vi "Load Manager Subpanel.vi"(8 "error in (no error)":errorcluster, 9 "Calling VI":refnum<vi>, 10 "Subpanel Type":T1, 11 "CIF_UI in":refnum<class "CIF_Manager_UI.lvclass">) -> (0 "error out":errorcluster, 2 "VI Reference":refnum<vi>, 3 "CIF_UI out":refnum<class "CIF_Manager_UI.lvclass">)   [LabVIEW 2021, in "CIF_Manager_UI.lvclass"]
uses:
  CIF_Manager_UI.lvclass
  C:/Program Files/National Instruments/LabVIEW 2021/vi.lib/CIF Foundation/CIF Core/CIFUI/CIF_UI.lvclass
  Typedef/Manager Subpanel Type.ctl
  <vilib>/CIF Foundation/CIF Core/CIFUI/CIF_UI.lvclass/CIF_UI.ctl
  CIF_Manager_UI.lvclass/CIF_Manager_UI.ctl
  Typedef/Class Data for Manager SubPanel.ctl
  <vilib>/CIF Foundation/CIF Core/CIFUI/Typedef/Class Data for SubPanel.ctl
  <vilib>/CIF Foundation/CIF Core/CIFUI/Typedef/Core UI References.ctl
  <vilib>/CIF Foundation/CIF Core/CIFUI/Typedef/SubPanel Events.ctl
  <vilib>/CIF Foundation/CIF Core/CIFUI/Typedef/New Connection Plugin Event Data.ctl
  Typedef/Core Manager UI References.ctl
  CIFPluginManager/typedef/New Connection Event Data.ctl
  <vilib>/gRPC/LabVIEW gRPC Library/Shared/grpcId.ctl
  <vilib>/CIF Foundation/CIF Core/CIFUI/Typedef/Subpanel Data.ctl
  <vilib>/CIF Foundation/CIF Core/CIFUI/Typedef/Plugin Subpanel Events.ctl
  <vilib>/CIF Foundation/CIF Core/CIFCore/Common/Typedef/Errors.ctl
  <vilib>/CIF Foundation/CIF Core/CIFUI/Accessors/Read Manager Connection.vi
  <vilib>/CIF Foundation/CIF Core/CIFUI/Accessors/Read Manager gRPC ID.vi
  <vilib>/CIF Foundation/CIF Core/CIFCore/Common/Utilities/Add Error Core.vi
  <vilib>/Utility/LVLibp/NI_PackedLibraryUtility.lvlib
  78e05929-4a52-4a7a-a51a-d61806b701c4.vi
  <vilib>/CIF Foundation/CIF Core/CIFCore/Common/CIFCoreCommon.lvlib
  <vilib>/CIF Foundation/CIF Core/CIFUtilities/CIFConfigurationFile/typedef/Location Type.ctl
  <vilib>/CIF Foundation/CIF Core/CIFUtilities/CIFConfigurationFile/CIF Configuration File.lvlib
  <vilib>/CIF Foundation/CIF Core/CIFUI/CIF_UI.lvclass
  <vilib>/gRPC/LabVIEW gRPC Library/grpc-lvsupport-release.lvlib
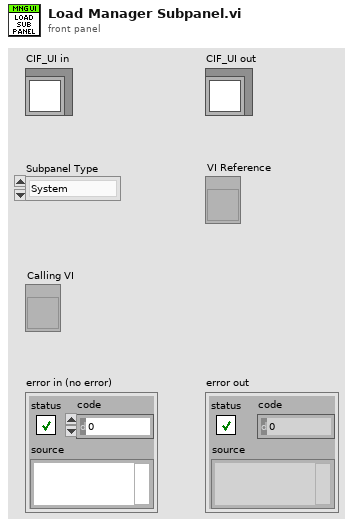
[diagram p1: front panel]
types:
  T1 = typedef "CIF_Manager_UI.lvclass/Manager Subpanel Type.ctl" = enum16{"System", "Errors", "Channel", "Plugin"}
  T2 = typedef "CIF_Manager_UI.lvclass/Class Data for Manager SubPanel.ctl" = cluster{"Class Data for SubPanel":T3, "Manager UI References":T6, "New Manager Connection":refnum<user-event>, "Manager gRPC ID":T7, "Manager Connection":bool}
  T3 = typedef "CIF_UI.lvclass/Class Data for SubPanel.ctl" = cluster{"IP Address":string, "Server Certificate File (.crt)":path, "Connected":bool, "Core UI References":T4, "Subpanel Events":T5, "Manager gRPC Port":u16}
  T4 = typedef "CIF_UI.lvclass/Core UI References.ctl" = cluster{"Plugin Status":refnum<vi>, "Plugin Status Valid":bool, "Connection":refnum<vi>, "Connection Valid":bool, "Exit":refnum<vi>, "Exit Valid":bool, "Run Listen":refnum<vi>, "Run Listen Valid":bool, "Clear Local Error":refnum<vi>, "Clear Local Error Valid":bool, "Local Error":refnum<vi>, "Local Error Valid":bool}
  T5 = typedef "CIF_UI.lvclass/SubPanel Events.ctl" = cluster{"Clear Local Error":refnum<user-event>, "Shutdown":refnum<user-event>, "Plugin Connection":refnum<user-event>}
  T6 = typedef "CIF_Manager_UI.lvclass/Core Manager UI References.ctl" = cluster{"Discovered Plugins":refnum<vi>, "Discovered Plugins Valid":bool, "Loaded Plugins":refnum<vi>, "Loaded Plugins Valid":bool, "Publisher Channels":refnum<vi>, "Publisher Channels Valid":bool, "Subscriber Channels":refnum<vi>, "Subscriber Channels Valid":bool, "Channel Connection":refnum<vi>, "Channel Connection Valid":bool, "New Plugin Load":refnum<vi>, "New Plugin Load Valid":bool, "Errors":refnum<vi>, "Errors Valid":bool, "Plugin to Abort":refnum<vi>, "Plugin to Abort Valid":bool, "CIF Manager Tab":refnum<vi>, "Manger Tab Valid":bool, "System Errors":refnum<vi>, "System Errors Valid":bool, "Plugin Selection":refnum<vi>, "Plugin Selection Valid":bool}
  T7 = typedef "grpc-lvsupport-release.lvlib/grpcId.ctl" = u64
  T8 = typedef "CIF_UI.lvclass/Subpanel Data.ctl" = cluster{"VI Reference":refnum<vi>, "Plugin Subpanel Events":T9}
  T9 = typedef "CIF_UI.lvclass/Plugin Subpanel Events.ctl" = cluster{"Plugin Shutdown":refnum<user-event>}
  T10 = typedef "CIFCoreCommon.lvlib/Errors.ctl" = enum8{"Invalid Clock ID", "Long Sleep", "gRPC Server Not Found", "Config Parse", "Timestamp Wrap", "Delayed Execution", "Duplicate Channel", "Missing Channel", "Incorrect Type", "Flatten Error", "Unflatten Data", "Unique Name", "Plugin Not Found", "Plugin Type Not Found", "Plugin Version Not Found", "Manager Not Found", "Numerical Issue", "Time Jump", "Clock ID Match", "Channel Length", "Plugin Connection", "gRPC Server Connection", "PPL Name Match", "Build", "Config Log Parse", "Plugin Load", "UI Subpanel Load", "Python Name", "Invalid Name", "Unable to Change Ch Buffer", "Failed Kill", "Failed SysExec", "Function Not Implemented", "Load Timeout", "Invalid FTE", "Manager Crash"}
  T11 = typedef "CIF Configuration File.lvlib/Location Type.ctl" = enum8{"Config File", "Manager", "Protos", "Plugins", "UI Plugins", "Logs", "Orchestrations", "Loaders"}
  T12 = typedef "CIF_Manager_UI.lvclass/Manager Subpanel Map.ctl" = map{T1, T8}
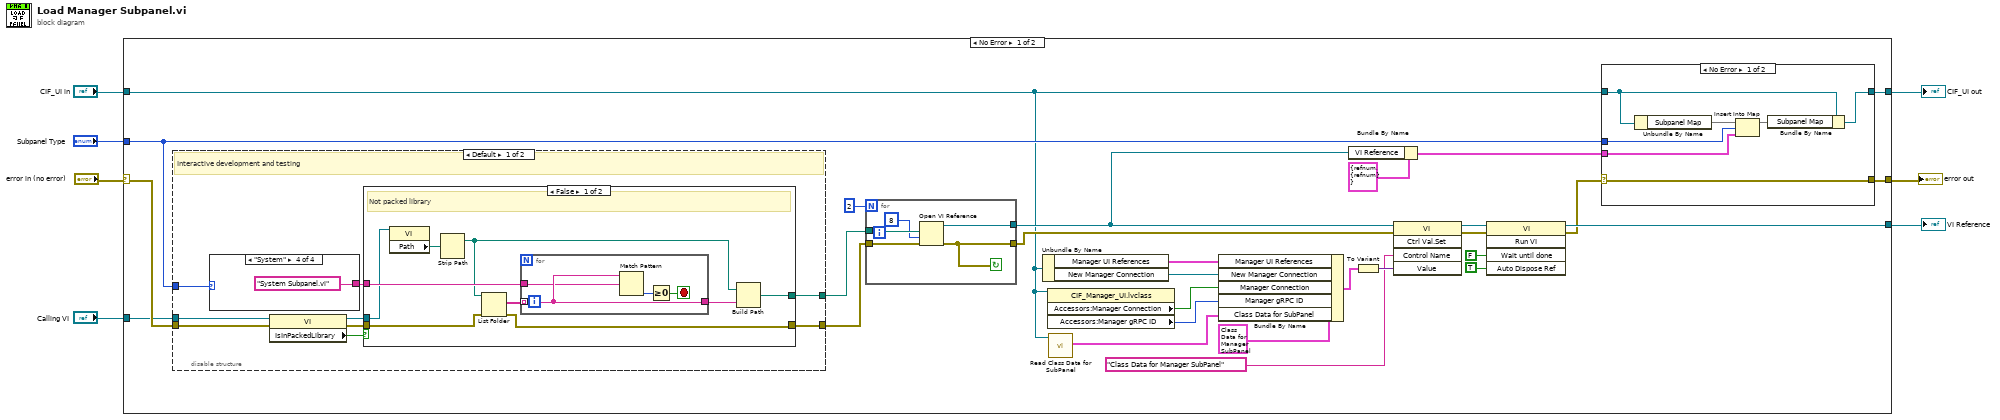
[diagram p0: block diagram]
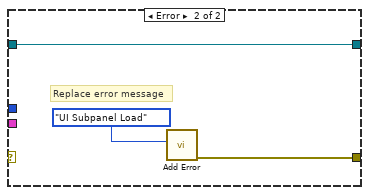
[diagram p2: hidden frame]
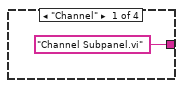
[diagram p3: hidden frame]
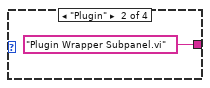
[diagram p4: hidden frame]
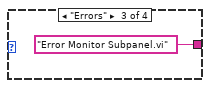
[diagram p5: hidden frame]
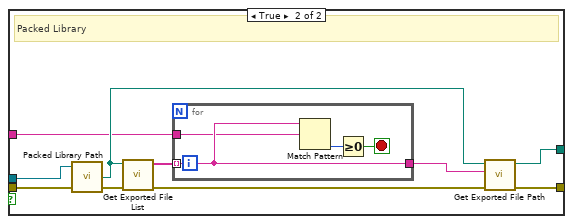
[diagram p6: hidden frame]
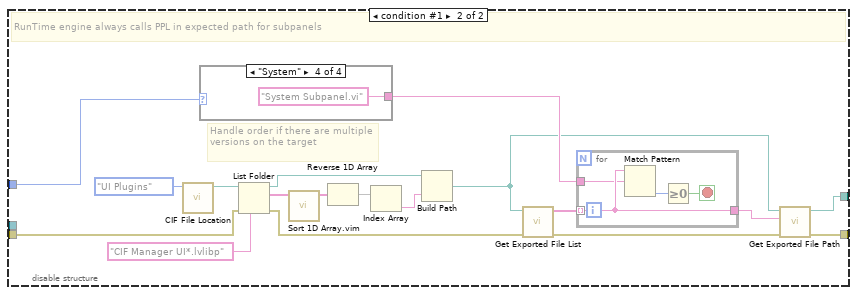
[diagram p7: hidden frame]
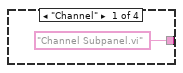
[diagram p8: hidden frame]
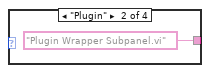
[diagram p9: hidden frame]
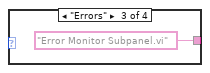
[diagram p10: hidden frame]
diagram:
  n1 = case shown="No Error" "error in (no error)" {
    selector: "error in (no error)" -> [w23 w118]
    tunnel: [w18 w118] -> w6
    tunnel: [w26 w117] -> w4
    tunnel: "CIF_UI in" -> [w12 w117]
    tunnel: "Subpanel Type" -> [w20 _]
    tunnel: [w25 _] -> w2
    tunnel: "Calling VI" -> [w19 _]
    frame No Error {
      n2 = disable-structure shown="Default" {
        disable-tunnel: w23 -> [w51 w90]
        disable-tunnel: [w50 w103] -> w22
        disable-tunnel: [w49 w102] -> w21
        disable-tunnel: w20 -> [w47 w86]
        disable-tunnel: w19 -> [w46 _]
        frame condition #0 (active) {
          # "Interactive development and testing"
          n3 = case shown="\"System\"" w47 {
            tunnel: ["Channel Subpanel.vi" ("regular expression") "Plugin Wrapper Subpanel.vi" ("regular expression") "Error Monitor Subpanel.vi" ("regular expression") "System Subpanel.vi" ("regular expression")] -> w48
            frame "Channel" {
            }
            frame "Plugin" {
            }
            frame "Errors" {
            }
            frame "System" {
            }
          }
          n4 = property class="VI"(reference=w46, error in=w51) -> (reference out=w53:refnum<vi>, error out=w54:errorcluster, "IsInPackedLibrary"=w52:bool)
          n5 = case shown="False" w52 {
            tunnel: w53 -> [w61 w81]
            tunnel: w54 -> [w65 w80]
            tunnel: [w59 w72] -> w49
            tunnel: [w64 w74] -> w50
            tunnel: w48 -> [w66 w73]
            frame False {
              # "Not packed library"
              n6 = property class="VI"(reference=w61) -> ("Path"=w62:path)  [unwired: 1 in, 2 out]
              n7 = Strip Path(path=w62) -> (stripped path=w63:path)  [unwired: 1 out]
              n8 = List Folder(path=w63, error in=w65) -> (filenames=w67:string[], error out=w64:errorcluster)  [unwired: 2 in, 2 out]
              n9 = for {
                tunnel: w67 -> [w69] mode=indexing
                tunnel: [w69] -> w60
                tunnel: w66 -> [w68]
                stop <- w70 stop-if-true
                n10 = Match Pattern(string=w69, regular expression=w68) -> (offset past match=w71:i32)  [unwired: 1 in, 3 out]
                n11 = Greater Or Equal To 0?(x=w71) -> (x >= 0?=w70:bool)
              }
              n12 = Build Path(base path=w63, name or relative path=w60) -> (appended path=w59:path)
            }
            frame True {
              # "Packed Library"
              n13 = call <vilib>:"Packed Library Path.vi"("error in (no error)"=w80, "vi reference"=w81) -> ("error out"=w75:errorcluster, "packed library path"=w76:path)  [unwired: 1 in, 1 out]
              n14 = call <vilib>:"Get Exported File List.vi"("error in (no error)"=w75, "packed library path"=w76) -> ("error out"=w78:errorcluster, "qualified names"=w77:string[])  [unwired: 7 in, 1 out]
              n15 = for {
                tunnel: w77 -> [w83] mode=indexing
                tunnel: [w83] -> w79
                tunnel: w73 -> [w82]
                stop <- w84 stop-if-true
                n16 = Match Pattern(string=w83, regular expression=w82) -> (offset past match=w85:i32)  [unwired: 1 in, 3 out]
                n17 = Greater Or Equal To 0?(x=w85) -> (x >= 0?=w84:bool)
              }
              n18 = call <vilib>:"Get Exported File Path.vi"("error in (no error)"=w78, "qualified name"=w79, "packed library path"=w76) -> ("error out"=w74:errorcluster, "path"=w72:path)  [unwired: 7 in]
            }
          }
        }
        frame condition #1 {
          # "Handle order if there are multiple versions on the target"
          # "RunTime engine always calls PPL in expected path for subpanels"
          n19 = call <vilib>:"CIF File Location.vi"("LocationType"=Location_Type."UI Plugins") -> ("Location"=w87:path)  [unwired: 10 in]
          n20 = case shown="\"System\"" w86 {
            tunnel: ["Channel Subpanel.vi" ("regular expression") "Plugin Wrapper Subpanel.vi" ("regular expression") "Error Monitor Subpanel.vi" ("regular expression") "System Subpanel.vi" ("regular expression")] -> w101
            frame "Channel" {
            }
            frame "Plugin" {
            }
            frame "Errors" {
            }
            frame "System" {
            }
          }
          n21 = List Folder(path=w87, pattern="CIF Manager UI*.lvlibp", error in=w90) -> (path out=w96:path, filenames=w93:string[], error out=w89:errorcluster)  [unwired: 1 in, 1 out]
          n22 = call "Sort 1D Array.vim"("unsorted array"=w93) -> ("sorted array"=w94:string[])  [unwired: 10 in]
          n23 = Reverse 1D Array(array=w94) -> (reversed array=w95:string[])
          n24 = Index Array(array=w95) -> (element=w97:string)  [unwired: 1 in]
          n25 = Build Path(base path=w96, name or relative path=w97) -> (appended path=w91:path)
          n26 = call <vilib>:"Get Exported File List.vi"("error in (no error)"=w89, "packed library path"=w91) -> ("error out"=w99:errorcluster, "qualified names"=w98:string[])  [unwired: 7 in, 1 out]
          n27 = for {
            tunnel: w98 -> [w105] mode=indexing
            tunnel: [w105] -> w100
            tunnel: w101 -> [w104]
            stop <- w106 stop-if-true
            n28 = Match Pattern(string=w105, regular expression=w104) -> (offset past match=w107:i32)  [unwired: 1 in, 3 out]
            n29 = Greater Or Equal To 0?(x=w107) -> (x >= 0?=w106:bool)
          }
          n30 = call <vilib>:"Get Exported File Path.vi"("error in (no error)"=w99, "qualified name"=w100, "packed library path"=w91) -> ("error out"=w103:errorcluster, "path"=w102:path)  [unwired: 7 in]
        }
      }
      n31 = for {
        N: 2 -> [_]
        tunnel: w21 -> [w116]
        tunnel: [w115] -> w24
        tunnel: [w112] -> w32
        tunnel: w22 -> [w114]
        stop <- w112 continue-if-true
        n32 = Open VI Reference(vi path=w116, options=8, error in (no error)=w114) -> (vi reference=w115:refnum<vi>, error out=w112:errorcluster)  [unwired: 3 in]
      }
      n33 = Unbundle By Name(w12) -> ("Manager UI References"=w14:T6, "New Manager Connection"=w11:refnum<user-event>)
      n34 = property class="CIF_Manager_UI.lvclass"(reference=w12) -> ("Accessors:Manager Connection"=w10:bool, "Accessors:Manager gRPC ID"=w9:T7)  [unwired: 1 in, 2 out]
      n35 = call <vilib>:"Read Class Data for SubPanel.vi"("CIF_UI in"=w12) -> ("Class Data for SubPanel"=w8:T3)  [unwired: 8 in, 2 out]
      n36 = Bundle By Name(cluster=T2 {"Class Data for SubPanel"={"IP Address"="", "Server Certificate File (.crt)"=path "", "Connected"=FALSE, "Core UI References"={"Plugin Status"=refnum, "Plugin Status Valid"=FALSE, "Connection"=refnum, "Connection Valid"=FALSE, "Exit"=refnum, "Exit Valid"=FALSE, "Run Listen"=refnum, "Run Listen Valid"=FALSE, "Clear Local Error"=refnum, "Clear Local Error Valid"=FALSE, "Local Error"=refnum, "Local Error Valid"=FALSE}, "Subpanel Events"={"Clear Local Error"=refnum, "Shutdown"=refnum, "Plugin Connection"=refnum}, "Manager gRPC Port"=0}, "Manager UI References"={"Discovered Plugins"=refnum, "Discovered Plugins Valid"=FALSE, "Loaded Plugins"=refnum, "Loaded Plugins Valid"=FALSE, "Publisher Channels"=refnum, "Publisher Channels Valid"=FALSE, "Subscriber Channels"=refnum, "Subscriber Channels Valid"=FALSE, "Channel Connection"=refnum, "Channel Connection Valid"=FALSE, "New Plugin Load"=refnum, "New Plugin Load Valid"=FALSE, "Errors"=refnum, "Errors Valid"=FALSE, "Plugin to Abort"=refnum, "Plugin to Abort Valid"=FALSE, "CIF Manager Tab"=refnum, "Manger Tab Valid"=FALSE, "System Errors"=refnum, "System Errors Valid"=FALSE, "Plugin Selection"=refnum, "Plugin Selection Valid"=FALSE}, "New Manager Connection"=refnum, "Manager gRPC ID"=0, "Manager Connection"=FALSE} ("Class Data for Manager SubPanel"), "Manager UI References"=w14, "New Manager Connection"=w11, "Manager Connection"=w10, "Manager gRPC ID"=w9, "Class Data for SubPanel"=w8) -> (w13:T2)
      n37 = Bundle By Name(cluster=T8 {"VI Reference"=refnum, "Plugin Subpanel Events"={"Plugin Shutdown"=refnum}} ("SubPanel Data"), "VI Reference"=w24) -> (w27:T8)
      n38 = To Variant(anything=w13) -> (Variant=w28:variant)
      n39 = invoke class="VI" method="Ctrl Val.Set"(reference=w24, error in=w32, "Control Name"="Class Data for Manager SubPanel", "Value"=w28) -> (reference out=w33:refnum<vi>, error out=w34:errorcluster)  [unwired: 1 in, 3 out]
      n40 = invoke class="VI" method="Run VI"(reference=w33, error in=w34, "Wait until done"=FALSE ("Wait Until Done"), "Auto Dispose Ref"=TRUE ("Auto Dispose Reference")) -> (reference out=w25:refnum<vi>, error out=w16:errorcluster)  [unwired: 1 in, 3 out]
      n41 = case shown="No Error" w16 {
        selector: w16 -> [w36 _]
        tunnel: w27 -> [w41 _]
        tunnel: [w39 w45] -> w26
        tunnel: w20 -> [w38 _]
        tunnel: [w36 w44] -> w18
        tunnel: w12 -> [w37 w45]
        frame No Error {
          n42 = Unbundle By Name(w37) -> ("Subpanel Map"=w42:T12)
          n43 = Insert Into Map(map in=w42, key=w38, value=w41) -> (map out=w40:T12)  [unwired: 2 out]
          n44 = Bundle By Name(cluster=w37, "Subpanel Map"=w40) -> (w39:refnum<class "CIF_Manager_UI.lvclass">)
        }
        frame Error {
          # "Replace error message"
          n45 = call <vilib>:"Add Error.vi"("Error"=Errors."UI Subpanel Load") -> ("error out"=w44:errorcluster)  [unwired: 10 in]
        }
      }
    }
    frame Error {
    }
  }
  "error out" <- w6
  "CIF_UI out" <- w4
  "VI Reference" <- w2
